vi "Cleanup.vi"(8 "error in (no error)":errorcluster, 11 "PlatformListPanel in":refnum<class "PlatformListPanel.lvclass">) -> (0 "error out":errorcluster)   [LabVIEW 2020, in "PicoG-App.lvlib" / "PlatformListPanel.lvclass"]
uses:
  PlatformListPanel.lvclass
  NavPanel/NavPanel.lvclass
  <vilib>/IlluminatedG/IG OOPanel/OOPanel/ArrayManager/ArrayManager.lvclass
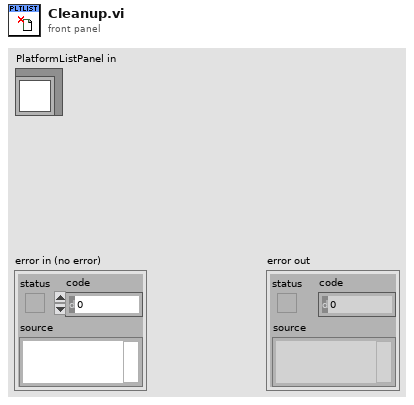
[diagram p1: front panel]
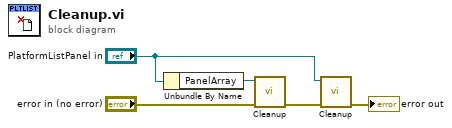
[diagram p0: block diagram]
diagram:
  n1 = Unbundle By Name("PlatformListPanel in") -> ("PanelArray"=w2:refnum<class "ArrayManager.lvclass">)
  n2 = call <vilib>:"Cleanup.vi"("error in (no error)"="error in (no error)", "PanelArray in"=w2) -> ("error out"=w1:errorcluster)  [unwired: 7 in, 2 out]
  n3 = call-parent <vilib>:"Cleanup.vi"("error in (no error)"=w1, "Panel in"="PlatformListPanel in") -> ("error out"=→"error out":errorcluster)  [unwired: 9 in]
